vi "MPM_DisConnect.vi"(8 "error in (no error)":errorcluster, 11 ".NET Reference in":refnum<k24>) -> (0 "error out":errorcluster, 3 "Reference out":refnum<k24>)   [LabVIEW 2017]
uses:
  D:/test/FULLband-sts/Fullband_Sample/DLL/InstrumentDLL.dll
  DLL/InstrumentDLL.dll
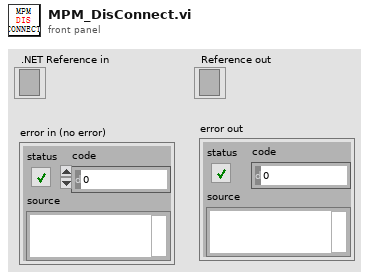
[diagram p1: front panel]
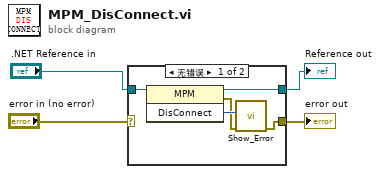
[diagram p0: block diagram]
diagram:
  n1 = case shown="无错误" "error in (no error)" {
    selector: "error in (no error)" -> [_ w11]
    tunnel: ".NET Reference in" -> [w9 w10]
    tunnel: [w8 w10] -> w3
    tunnel: [w5 w11] -> w2
    frame No Error {
      n2 = invoke on="调用节点" class="MPM" method="DisConnect"(reference=w9) -> (reference out=w8:refnum<k24>, error out=w6:errorcluster, "DisConnect"=w7:i32)  [unwired: 2 in]
      n3 = call "Show_Error.vi"("error in (no error)"=w6, "Error"=w7) -> ("error out"=w5:errorcluster)  [unwired: 9 in]
    }
    frame Error {
    }
  }
  "Reference out" <- w3
  "error out" <- w2
